vi "MTM2_acceptCommand_setValue.vi"(8 "error in (no error)":errorcluster, 11 "command_setValue_Ctl":T1={"private_rcvStamp"=0.0, "parametersAndValues"="                                                                                                                                                                                                                                                                "}) -> (0 "error out":errorcluster, 2 "function return":i32, 3 "command_setValue_Ctl out":T1={"private_rcvStamp"=0.0, "parametersAndValues"="                                                                                                                                                                                                                                                                "})   [LabVIEW 2018, in "SALLV_MTM2.lvlib"]
doc: "int MTM2_shm_acceptCommand_setValueLV(MTM2_command_setValueLV *command_setValue_Ctl );"
uses:
  DataTypes/command_setValue.ctl
  SALLV_MTM2.lvlib
  SALLV_MTM2.so
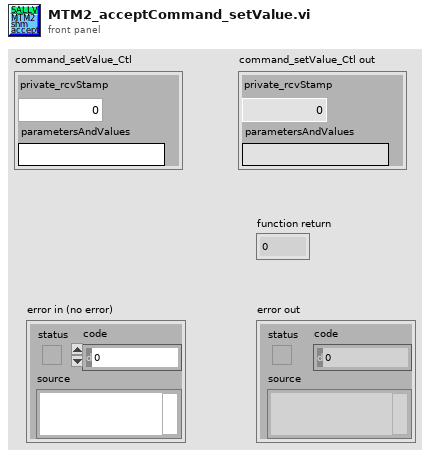
[diagram p1: front panel]
types:
  T1 = typedef "SALLV_MTM2.lvlib/command_setValue.ctl" = cluster{"private_rcvStamp":dbl, "parametersAndValues":string}
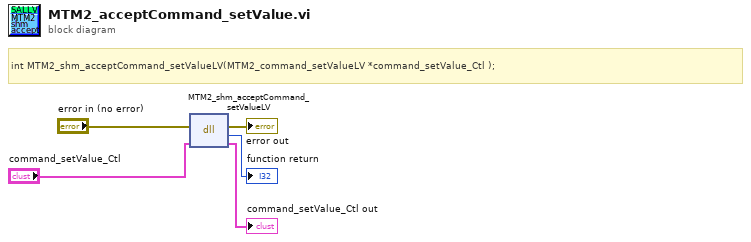
[diagram p0: block diagram]
diagram:
  # "int MTM2_shm_acceptCommand_setValueLV(MTM2_command_setValueLV *command_setValue_Ctl );"
  n1 = dll-call lib="home/ttsai/Documents/salTestLabViewApi/SALLV_MTM2/SALLV_MTM2.*" fn="MTM2_shm_acceptCommand_setValueLV"(error in="error in (no error)", "command_setValue_Ctl"="command_setValue_Ctl") -> (error out=→"error out":errorcluster, →"function return":i32, "command_setValue_Ctl"=→"command_setValue_Ctl out":T1)  [unwired: 2 in, 1 out]
